vi "subvi_Get_setting.vi"(8 "에러 입력(에러 없음)":errorcluster, 10 "Input adress":u16[](array[numeric])=[0, 10, 20], 11 "Modbus Master 입력":refnum<class "Modbus Master.lvclass">) -> (0 "에러 출력":errorcluster, 2 "register values":u16[](array[numeric]), 3 "Modbus Master 출력":refnum<class "Modbus Master.lvclass">)   [LabVIEW 2016]
uses:
  <vilib>/NI/Modbus Library/API/Master/Modbus Master.lvclass
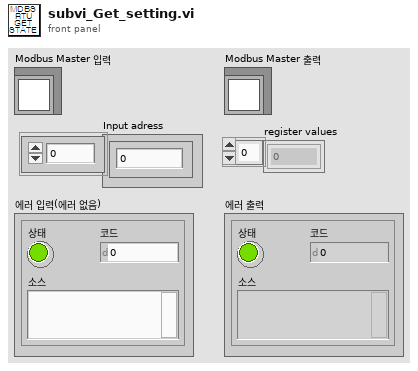
[diagram p1: front panel]
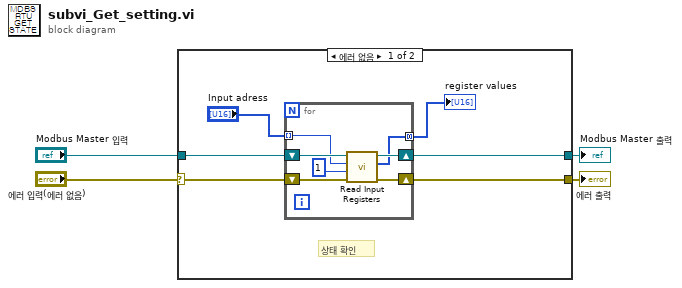
[diagram p0: block diagram]
diagram:
  n1 = case shown="에러 없음" "에러 입력(에러 없음)" {
    selector: "에러 입력(에러 없음)" -> [w5 w19]
    tunnel: "Modbus Master 입력" -> [w8 w18]
    tunnel: [w7 w19] -> w3
    tunnel: [w6 w18] -> w2
    frame No Error {
      # "상태 확인"
      n2 = for {
        shift-right: [w14] -> w7
        shift-left: w5 -> [w17]
        shift-right: [w15] -> w6
        shift-left: w8 -> [w13]
        tunnel: "Input adress" -> [w12] mode=indexing
        tunnel: [w11] -> w10 mode=concatenating
        n3 = call-dynamic "Read Input Registers.vi"("error in"=w17, "number of inputs"=u16 1, "starting address"=w12, "Modbus master in"=w13) -> ("error out"=w14:errorcluster, "register values"=w11:u16[], "Modbus master out"=w15:refnum<class "Modbus Master.lvclass">)  [unwired: 5 in]
      }
      "register values" <- w10
    }
    frame Error {
    }
  }
  "에러 출력" <- w3
  "Modbus Master 출력" <- w2
